vi "1,3 B Spoof Reality.vi"(11 "Simulator Bounds":T2={"Simulator E Range"=20.0, "Simulator E Min"=-10.0, "Simulator N Range"=20.0, "Simulator N Min"=-10.0}) -> (0 "Apparent Wind\nDirection":T5, 1 "Apparent Wind\nSpeed":T3, 2 "Robot velocity":T1 {"East" format="%#_5g"}, 3 "Robot\nHeading":T4 format="%05.1f", 4 "Boat Path":cluster{"X Position":dbl, "Y Position":dbl}[](array[cluster]), 5 "Robot UTM Location":T6 {"North" format="%#_10f"; "East" format="%#_8f"}, 6 "XY Graph":cluster{dbl, dbl}[](graph))   [LabVIEW 2011]
uses:
  2-Think/2 Typedefs/UTM Location.ctl
  2-Think/2 Typedefs/heading.ctl
  2-Think/2 Typedefs/apparent wind direction.ctl
  2-Think/2 Typedefs/apparent wind speed.ctl
  2-Think/2 Typedefs/Velocity.ctl
  1,3 B Typedefs/simulator bounds.ctl
  2-Think/2 Typedefs/pitch and roll.ctl
  2-Think/2 Typedefs/generalized sensor status.ctl
  2-Think/2 Typedefs/indicator LED.ctl
  2-Think/2 Typedefs/generalized actuator status.ctl
  2-Think/2 Globals/2 Global.vi
panel:
  in  "Absolute Water Current":T1 {"East" format="%#_5g"}
  out "Wind dV":T3
  out "Total Drag dV":dbl
  out "Rudder Drag":dbl
  in  "Rudder Drag Coefficient":dbl=1.5
  out "Speed":T3
  in  "Hull Drag Coefficient":dbl=0.3
  out "dHeading/dT":T4 format="%05.1f"
  out "Apparent Wind":cluster{"X Position":dbl, "Y Position":dbl}
  in  "Wind Direction":dbl=45.0
  in  "Wind Speed":dbl=2.0
  # "Add reasonable values to all of the things you can set here."
  # "This is the Bass. It's catchy. You like it."
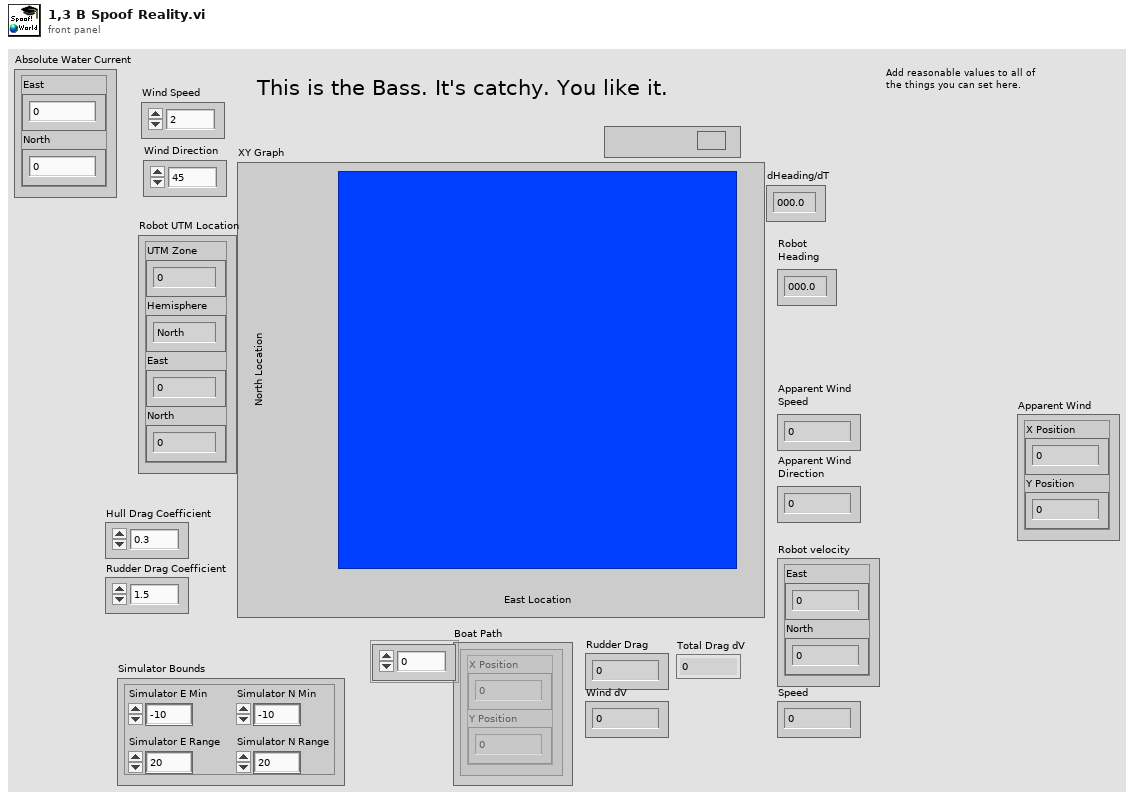
[diagram p1: front panel]
types:
  T1 = typedef "Velocity.ctl" = cluster{"East":dbl, "North":dbl}
  T2 = typedef "simulator bounds.ctl" = cluster{"Simulator E Range":dbl, "Simulator E Min":dbl, "Simulator N Range":dbl, "Simulator N Min":dbl}
  T3 = typedef "apparent wind speed.ctl" = dbl
  T4 = typedef "heading.ctl" = dbl
  T5 = typedef "apparent wind direction.ctl" = dbl
  T6 = typedef "UTM Location.ctl" = cluster{"UTM Zone":dbl, "Hemisphere":enum16{"North", "South"}, "East":dbl, "North":dbl}
  T7 = typedef "pitch and roll.ctl" = cluster{"Pitch":dbl, "Roll":dbl}
  T8 = typedef "generalized sensor status.ctl" = cluster{"Sensor Connected":T9, "Sensor Initialized":T9, "Sensor OK":T9, "Latest Error String":string, "GPS Lock":T9}
  T9 = typedef "indicator LED.ctl" = bool
  T10 = typedef "generalized actuator status.ctl" = cluster{"Actuator Connected":T9}
  T11 = typedef "robot velocity.ctl" = cluster{"East":dbl, "North":dbl}
  T12 = typedef "apparent wind.ctl" = cluster{"Toward Fore":dbl, "Toward Starboard":dbl}
  T13 = typedef "setpoints to boat.ctl" = cluster{"Sail Position":T14, "Rudder Angle":T15}
  T14 = typedef "sail setpt.ctl" = dbl
  T15 = typedef "rudder angle.ctl" = dbl
  T16 = typedef "rate of turn.ctl" = dbl
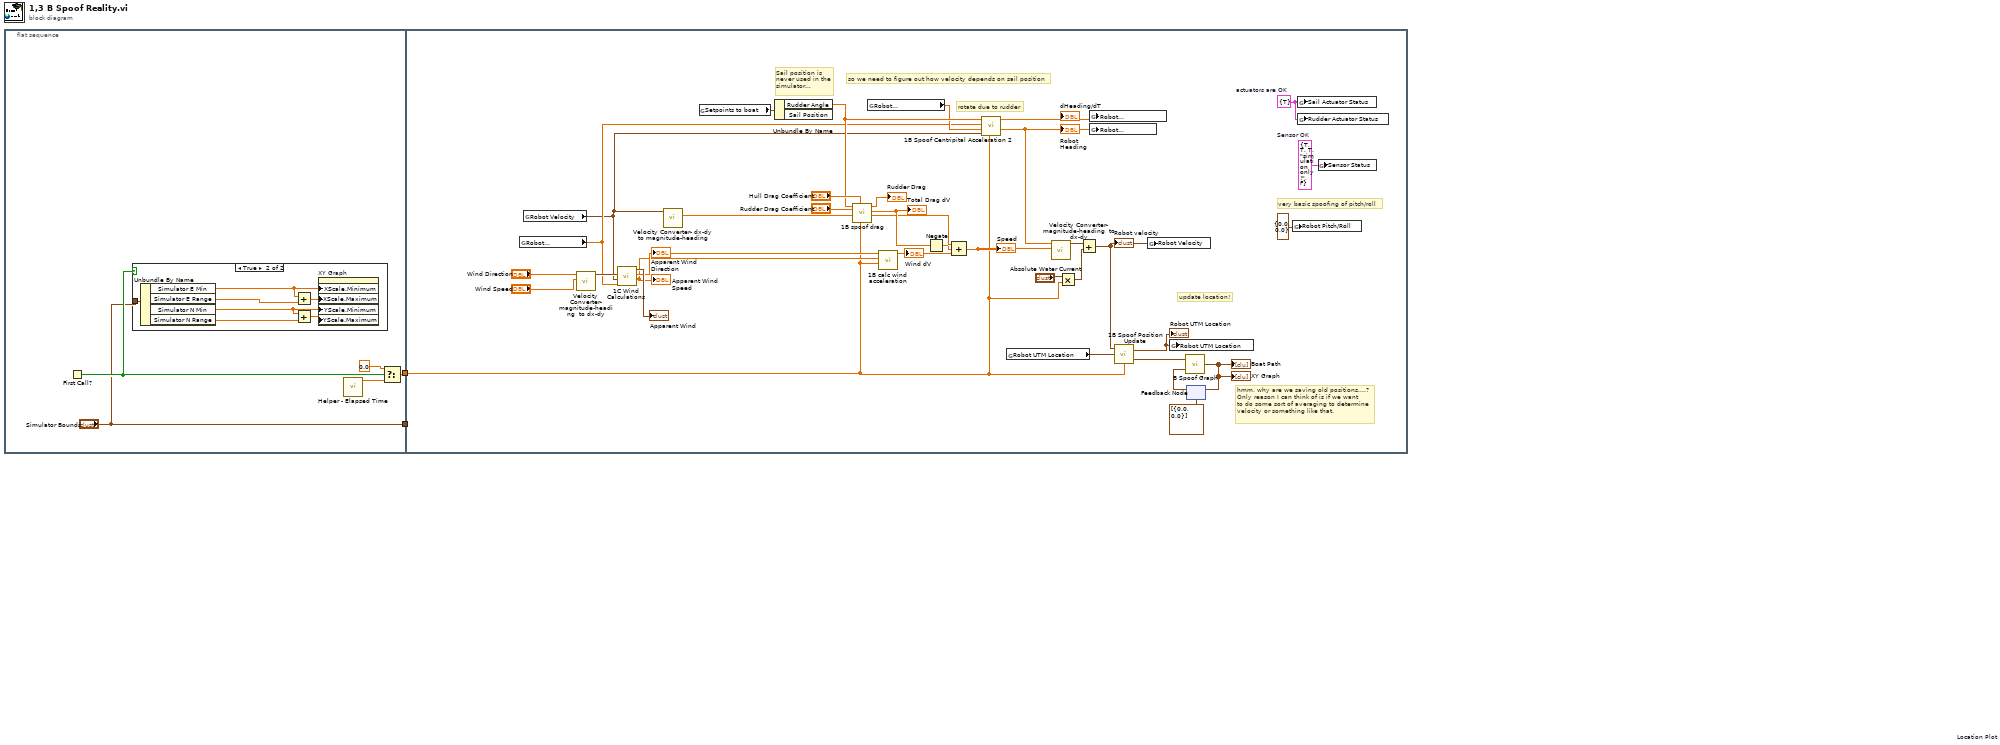
[diagram p0: block diagram]
diagram:
  n1 = flat-sequence {
    tunnel: [w7] -> w2
    tunnel: ["Simulator Bounds"] -> w1
    tunnel: w2 -> [w16]
    tunnel: w1 -> [_]
    frame #0 {
      n2 = First Call?() -> (First Call?: T/F=w6:bool)
      n3 = case shown="True" w6 {
        tunnel: "Simulator Bounds" -> [_ w14]
        frame False {
        }
        frame True {
          n4 = Unbundle By Name(w14) -> ("Simulator E Min"=w11:dbl, "Simulator E Range"=w10:dbl, "Simulator N Min"=w8:dbl, "Simulator N Range"=w9:dbl)
          n5 = Add(x=w11, y=w10) -> (x+y=w13:dbl)
          n6 = Add(x=w8, y=w9) -> (x+y=w12:dbl)
          n7 = property on="XY Graph" class="XYGraph (strict)"("XScale.Minimum"=w11, "XScale.Maximum"=w13, "YScale.Minimum"=w8, "YScale.Maximum"=w12) -> ()  [unwired: 2 in, 2 out]
        }
      }
      n8 = call "Helper - Elapsed Time.vi"() -> ("Time Elapsed (s)\nSince Last Iteration"=w4:dbl)  [unwired: 10 in, 1 out]
      n9 = Select(t=0.0 ("f"), s=w6, f=w4) -> (s? t:f=w7:dbl)
    }
    frame #1 {
      w44 = T8 {"Sensor Connected"=TRUE, "Sensor Initialized"=TRUE, "Sensor OK"=TRUE, "Latest Error String"="simulation only!", "GPS Lock"=FALSE}  # Sensor OK
      w45 = T10 {"Actuator Connected"=TRUE}  # actuators are OK
      # "so we need to figure out how velocity depends on sail position"
      # "Sail position is never used in the simulator..."
      # "hmm, why are we saving old positions....?\nOnly reason I can think of is if we want\nto do some sort of averaging to determine\nvelocity or something like that."
      # "rotate due to rudder"
      # "update location!"
      # "very basic spoofing of pitch/roll"
      n10 = global read "2 Global.vi" "Robot\nHeading"() -> (w24:T4)
      n11 = global read "2 Global.vi" "Robot Velocity"() -> (w23:T11)
      n12 = call "Velocity Converter- magnitude-heading  to dx-dy.vi"("Magnitude"="Wind Speed", "Heading"="Wind Direction") -> ("Vector Out"=w41:T1)  [unwired: 9 in]
      n13 = call "1C Wind Calculations.vi"("Boat Heading"=w24, "Boat Velocity"=w23, "Absolute Wind"=w41) -> ("Apparent Wind Speed"=w36:T3, "Apparent Wind\nDirection"=w37:T5, "Apparent Wind"=→"Apparent Wind":T12)  [unwired: 5 in]
      "Apparent Wind\nDirection" <- w37
      "Apparent Wind\nSpeed" <- w36
      n14 = call "Velocity Converter- dx-dy to magnitude-heading.vi"("Vector In"=w23) -> ("Magnitude Out"=w28:dbl)  [unwired: 9 in, 1 out]
      n15 = global read "2 Global.vi" "Setpoints to boat"() -> (w46:T13)
      n16 = Unbundle By Name(w46) -> ("Rudder Angle"=w32:T15)  [unwired: 1 out]
      n17 = call "1B spoof drag.vi"("time elapsed since last iteration"=w16, "Hull Drag Coefficient"="Hull Drag Coefficient", "Speed"=w28, "Rudder Drag Coefficient"="Rudder Drag Coefficient", "Rudder Angle"=w32) -> ("Total Drag dV"=w29:dbl, "Rudder Drag"=→"Rudder Drag":dbl)  [unwired: 5 in]
      "Total Drag dV" <- w29
      n18 = global read "2 Global.vi" "Robot\nRate of Turn"() -> (w25:T16)
      n19 = call "1B calc wind acceleration.vi"("time elapsed since last iteration"=w16, "Apparent Wind Speed in"=w36, "Apparent Wind\nDirection"=w37) -> ("Wind dV"=w26:T3)  [unwired: 8 in]
      "Wind dV" <- w26
      n20 = Negate(x=w29) -> (-x=w27:dbl)
      n21 = Compound Arithmetic op=ADD(w28, w27, w26) -> (w30:T3)
      "Speed" <- w30
      n22 = call "1B Spoof Centripital Acceleration 2.vi"("time elapsed since last iteration"=w16, "Robot Velocity"=w23, "dHeading/dT in"=w25, "Robot\nHeading in"=w24, "Rudder Angle"=w32) -> ("Robot\nHeading out"=w34:T4, "dHeading/dT"=w39:T4)  [unwired: 4 in, 1 out]
      "Robot\nHeading" <- w34
      "dHeading/dT" <- w39
      n23 = global read "2 Global.vi" "Robot UTM Location"() -> (w22:T6)
      n24 = call "Velocity Converter- magnitude-heading  to dx-dy.vi"("Magnitude"=w30, "Heading"=w34) -> ("Vector Out"=w20:T1)  [unwired: 9 in]
      n25 = Multiply(x="Absolute Water Current", y=w16) -> (x*y=w17:T1)
      n26 = Add(x=w20, y=w17) -> (x+y=w19:T1)
      "Robot velocity" <- w19
      n27 = global write "2 Global.vi" "Robot\nRate of Turn"(w39) -> ()
      n28 = global write "2 Global.vi" "Robot\nHeading"(w34) -> ()
      n29 = call "1B Spoof Position Update.vi"("dt"=w16, "Robot UTM Location"=w22, "Robot Velocity"=w19) -> ("XY position"=w15:cluster{"East":dbl, "North":dbl}, "New Robot UTM Location"=w21:T6)  [unwired: 1 in]
      "Robot UTM Location" <- w21
      n30 = global write "2 Global.vi" "Robot Velocity"(w19) -> ()
      n31 = global write "2 Global.vi" "Robot UTM Location"(w21) -> ()
      n32 = feedback #1 "Location Plot"(cluster{dbl, dbl}[] [{0.0, 0.0}] ("XY Graph")) -> (w47:cluster{dbl, dbl}[])
      n33 = call "B Spoof Graph.vi"("XY Graph"=w47, "New Position"=w15) -> ("Array"=w48:cluster{"X Position":dbl, "Y Position":dbl}[])
      "XY Graph" <- w48
      "Boat Path" <- w48
      n34 = feedback-in #1(w48) -> ()
      n35 = global write "2 Global.vi" "Robot Pitch/Roll"(T7 {"Pitch"=0.0, "Roll"=0.0} ("Robot Pitch/Roll")) -> ()
      n36 = global write "2 Global.vi" "Sail Actuator Status"(w45) -> ()
      n37 = global write "2 Global.vi" "Rudder Actuator Status"(w45) -> ()
      n38 = global write "2 Global.vi" "Sensor Status"(w44) -> ()
    }
  }
